vi "ILD from Array Data for S4p Tool.vi"(8 "Frequency":dbl[](array[numeric]), 9 "Data in":dbl[][](array[numeric]) caption="Data In" format="%0.3f", 10 "Data path":path caption="Data Save Path", 11 "Spec":enum16{"IEEE802.3ba", "FDR", "EDR"}(ring)) -> (1 "Data out":dbl[][](array[numeric]), 2 "ILD":cluster{"all rows":dbl[], sgl[]}[](graph), 3 "IL Fitted":cluster{"all rows":dbl[], "IL":dbl[]}[](graph))   [LabVIEW 2011]
uses:
  <vilib>/Analysis/baseanly.llb/Real A x B.vi
  <vilib>/Analysis/baseanly.llb/Real Inverse Matrix.vi
  <vilib>/Analysis/baseanly.llb/A x Vector.vi
  <vilib>/Utility/file.llb/Write To Spreadsheet File (DBL).vi
  <vilib>/Analysis/NI_AALBase.lvlib
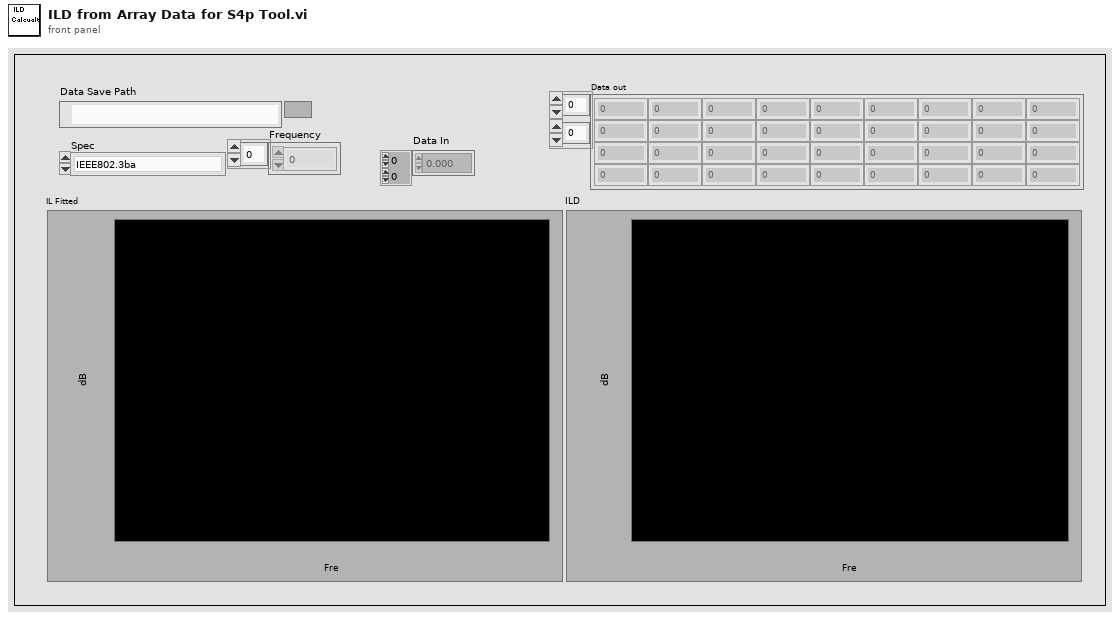
[diagram p1: front panel]
types:
  T1 = typedef "NI_Matrix.lvlib/RealMatrix.ctl" = dbl[][]
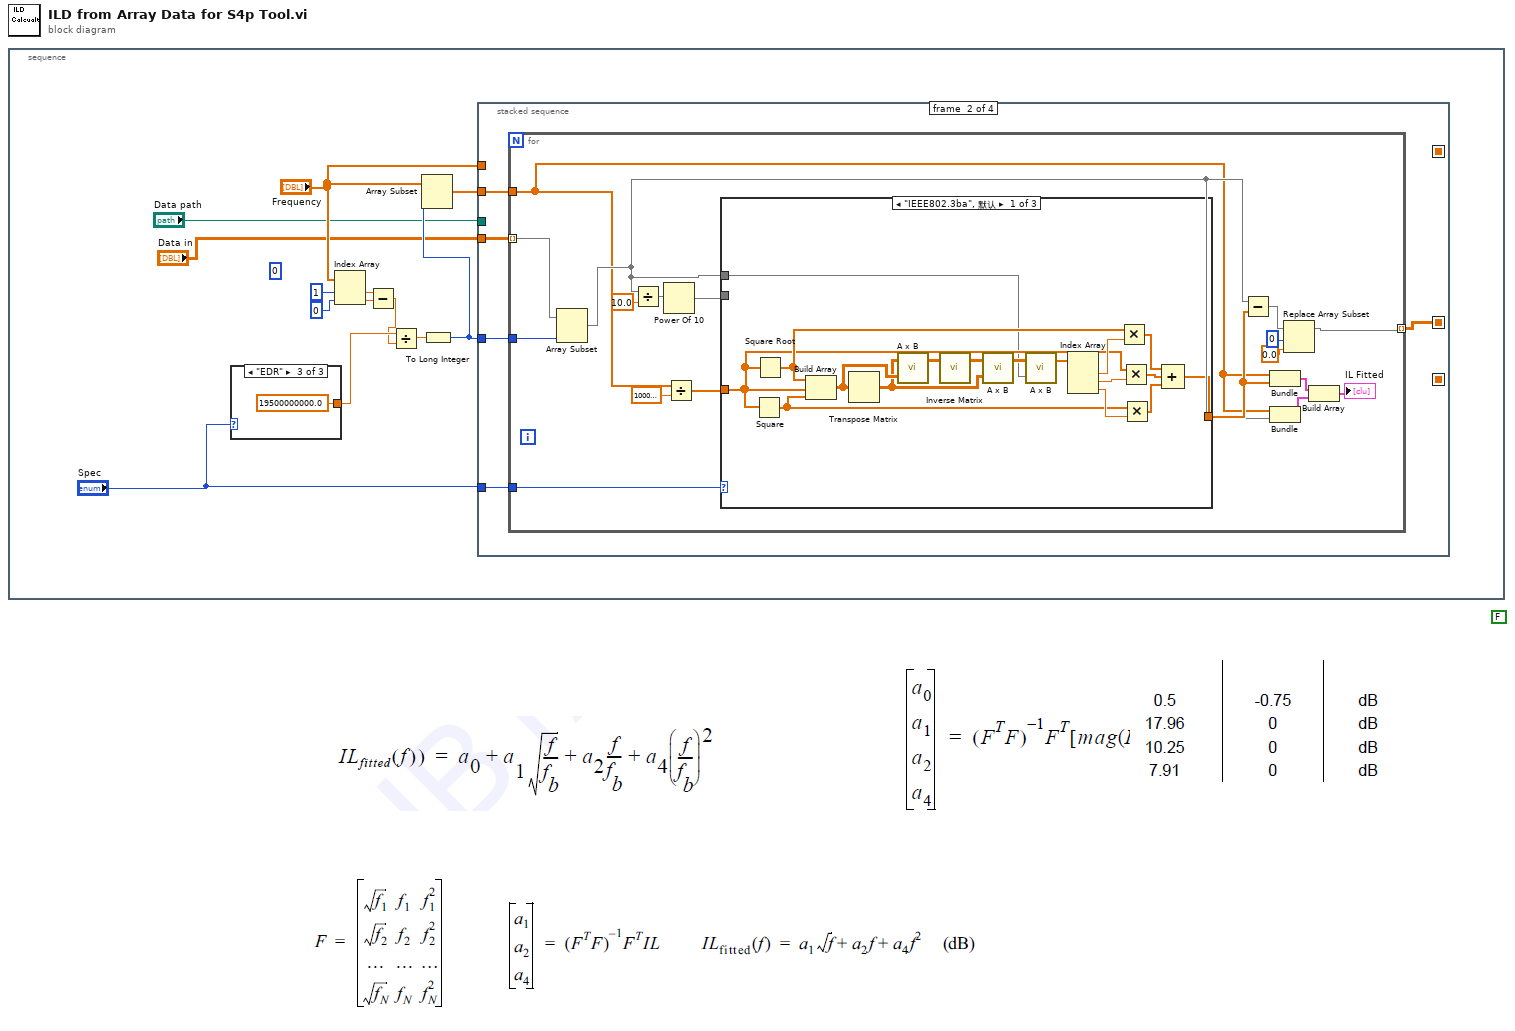
[diagram p0: block diagram]
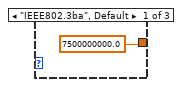
[diagram p2: hidden frame]
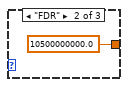
[diagram p3: hidden frame]
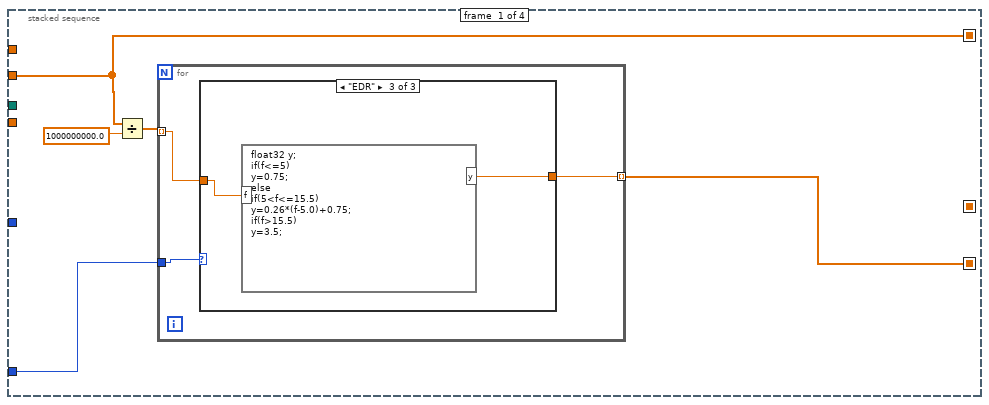
[diagram p4: hidden frame]
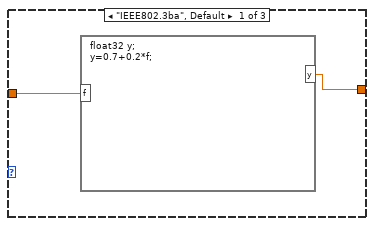
[diagram p5: hidden frame]
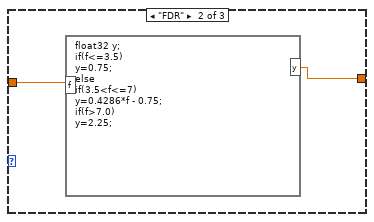
[diagram p6: hidden frame]
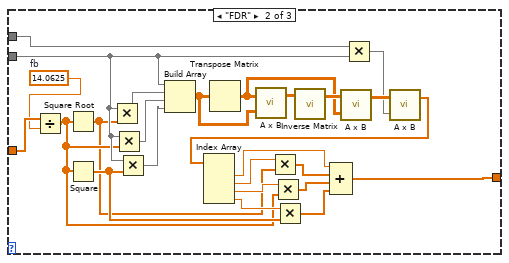
[diagram p7: hidden frame]
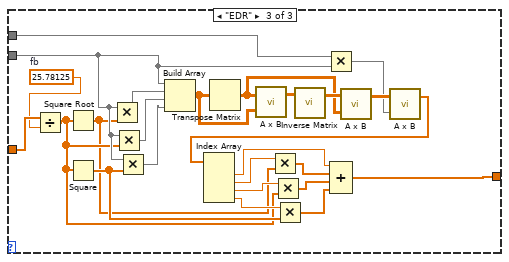
[diagram p8: hidden frame]
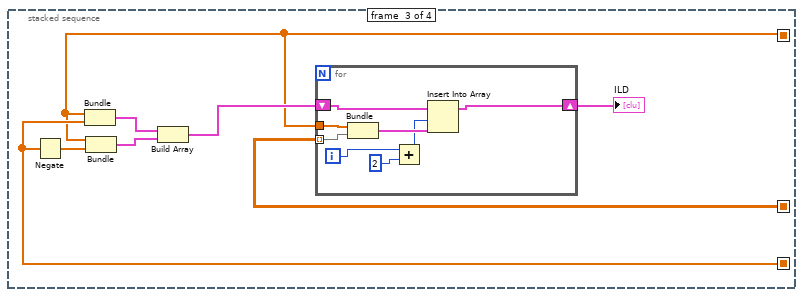
[diagram p9: hidden frame]
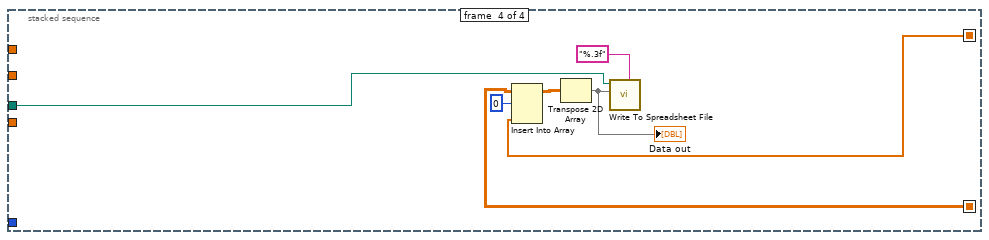
[diagram p10: hidden frame]
diagram:
  (unwired) FALSE
  n1 = stacked-sequence {
    frame #0 {
      (unwired) 0 ("禁用的索引 (列)")
      n2 = case shown="\"EDR\"" "Spec" {
        tunnel: [7500000000.0 ("y") 10500000000.0 ("y") 19500000000.0 ("y")] -> w10
        frame "IEEE802.3ba", Default {
        }
        frame "FDR" {
        }
        frame "EDR" {
        }
      }
      n3 = Index Array(array="Frequency", index #1=1 ("索引"), index #2=0 ("索引")) -> (element #1=w8:dbl, element #2=w9:dbl)
      n4 = Subtract(x=w8, y=w9) -> (x-y=w7:dbl)
      n5 = Divide(x=w10, y=w7) -> (x/y=w6:dbl)
      n6 = To Long Integer(number=w6) -> (32bit integer=w4:i32)
      n7 = Array Subset(array="Frequency", length=w4) -> (w5:dbl[])  [unwired: 1 in]
      n8 = stacked-sequence {
        seq-local: [w20 _ _ _] -> [_ _ w126 _]
        seq-local: [w17 _ _ _] -> [_ _ w122 w140]
        seq-local: [_ w33 _ _] -> [_ _ w123 w141]
        tunnel: "Data in" -> [_ w35 _ _]
        tunnel: "Spec" -> [w21 w34 _ _]
        tunnel: w5 -> [w17 w32 _ _]
        tunnel: "Data path" -> [_ _ _ w137]
        tunnel: w4 -> [_ w31 _ _]
        tunnel: "Frequency" -> [_ _ _ _]
        frame #0 {
          n9 = Divide(x=w17, y=1000000000.0) -> (x/y=w19:dbl[])
          n10 = for {
            tunnel: w21 -> [w24]
            tunnel: w19 -> [w23] mode=indexing
            tunnel: [w22] -> w20 mode=indexing
            n11 = case shown="\"EDR\"" w24 {
              tunnel: w23 -> [w26 w28 w30]
              tunnel: [w25 w27 w29] -> w22
              frame "IEEE802.3ba", Default {
                n12 = formula code="float32 y;\ny=0.7+0.2*f;"("f"=w26) -> ("y"=w25:sgl)
              }
              frame "FDR" {
                n13 = formula code="float32 y;\nif(f<=3.5)\ny=0.75;\nelse\nif(3.5<f<=7)\ny=0.4286*f - 0.75;\nif(f>7.0)\ny=2.25;"("f"=w28) -> ("y"=w27:sgl)
              }
              frame "EDR" {
                n14 = formula code="float32 y;\nif(f<=5)\ny=0.75;\nelse\nif(5<f<=15.5)\ny=0.26*(f-5.0)+0.75;\nif(f>15.5)\ny=3.5;"("f"=w30) -> ("y"=w29:sgl)
              }
            }
          }
        }
        frame #1 {
          n15 = for {
            tunnel: w35 -> [w36] mode=indexing
            tunnel: [w45] -> w33 mode=indexing
            tunnel: w34 -> [w44]
            tunnel: w32 -> [w37]
            tunnel: w31 -> [w39]
            n16 = Array Subset(array=w36, length=w39) -> (w38:dbl[])  [unwired: 1 in]
            n17 = Divide(x=w38, y=10.0 ("新元素/子数组")) -> (x/y=w42:dbl[])
            n18 = Power Of 10(x=w42) -> (10^x=w41:dbl[])
            n19 = Divide(x=w37, y=1000000000.0) -> (x/y=w40:dbl[])
            n20 = case shown="\"IEEE802.3ba\", 默认" w44 {
              tunnel: [w56 w71 w96] -> w49
              tunnel: w40 -> [w55 w95 w120]
              tunnel: w38 -> [w54 w85 w110]
              tunnel: w41 -> [_ w84 w109]
              frame "IEEE802.3ba", Default {
                n21 = Square(x=w55) -> (x^2=w60:dbl[])
                n22 = Square Root(x=w55) -> (sqrt(x)=w61:dbl[])
                n23 = Build Array(w61, w55, w60) -> (w70:T1)
                n24 = Transpose Matrix(1:w70) -> (0:w68:T1)
                n25 = call-poly <vilib>:"A x B.vi"("B"=w70, "A"=w68) -> ("A x B"=w69:T1)  [unwired: 1 out]
                n26 = call-poly <vilib>:"Inverse Matrix.vi"("Input Matrix"=w69) -> ("Inverse Matrix"=w67:T1)  [unwired: 1 in, 1 out]
                n27 = call-poly <vilib>:"A x B.vi"("B"=w68, "A"=w67) -> ("A x B"=w66:T1)  [unwired: 1 out]
                n28 = call-poly <vilib>:"A x B.vi"("Vector"=w54, "A"=w66) -> ("A x Vector"=w65:dbl[])  [unwired: 1 out]
                n29 = Index Array(array=w65) -> (element #1=w62:dbl, element #2=w63:dbl, element #3=w64:dbl)  [unwired: 3 in]
                n30 = Multiply(x=w61, y=w62) -> (x*y=w59:dbl[])
                n31 = Multiply(x=w55, y=w63) -> (x*y=w58:dbl[])
                n32 = Multiply(x=w60, y=w64) -> (x*y=w57:dbl[])
                n33 = Compound Arithmetic op=ADD(w59, w58, w57) -> (w56:dbl[])
              }
              frame "FDR" {
                w94 = 14.0625  # fb
                n34 = Divide(x=w95, y=w94) -> (x/y=w73:dbl[])
                n35 = Square Root(x=w73) -> (sqrt(x)=w72:dbl[])
                n36 = Square(x=w73) -> (x^2=w74:dbl[])
                n37 = Multiply(x=w84, y=w72) -> (x*y=w93:dbl[])
                n38 = Multiply(x=w84, y=w73) -> (x*y=w92:dbl[])
                n39 = Multiply(x=w84, y=w74) -> (x*y=w91:dbl[])
                n40 = Build Array(w84, w93, w92, w91) -> (w90:T1)
                n41 = Transpose Matrix(1:w90) -> (0:w87:T1)
                n42 = call-poly <vilib>:"A x B.vi"("B"=w90, "A"=w87) -> ("A x B"=w89:T1)  [unwired: 1 out]
                n43 = call-poly <vilib>:"Inverse Matrix.vi"("Input Matrix"=w89) -> ("Inverse Matrix"=w88:T1)  [unwired: 1 in, 1 out]
                n44 = call-poly <vilib>:"A x B.vi"("B"=w87, "A"=w88) -> ("A x B"=w86:T1)  [unwired: 1 out]
                n45 = Multiply(x=w85, y=w84) -> (x*y=w83:dbl[])
                n46 = call-poly <vilib>:"A x B.vi"("Vector"=w83, "A"=w86) -> ("A x Vector"=w82:dbl[])  [unwired: 1 out]
                n47 = Index Array(array=w82) -> (element #1=w81:dbl, element #2=w80:dbl, element #3=w79:dbl, element #4=w78:dbl)  [unwired: 4 in]
                n48 = Multiply(x=w80, y=w72) -> (x*y=w77:dbl[])
                n49 = Multiply(x=w79, y=w73) -> (x*y=w76:dbl[])
                n50 = Multiply(x=w78, y=w74) -> (x*y=w75:dbl[])
                n51 = Compound Arithmetic op=ADD(w81, w77, w76, w75) -> (w71:dbl[])
              }
              frame "EDR" {
                w119 = 25.78125  # fb
                n52 = Divide(x=w120, y=w119) -> (x/y=w98:dbl[])
                n53 = Square Root(x=w98) -> (sqrt(x)=w97:dbl[])
                n54 = Square(x=w98) -> (x^2=w99:dbl[])
                n55 = Multiply(x=w109, y=w97) -> (x*y=w118:dbl[])
                n56 = Multiply(x=w109, y=w98) -> (x*y=w117:dbl[])
                n57 = Multiply(x=w109, y=w99) -> (x*y=w116:dbl[])
                n58 = Build Array(w109, w118, w117, w116) -> (w115:T1)
                n59 = Transpose Matrix(1:w115) -> (0:w112:T1)
                n60 = call-poly <vilib>:"A x B.vi"("B"=w115, "A"=w112) -> ("A x B"=w114:T1)  [unwired: 1 out]
                n61 = call-poly <vilib>:"Inverse Matrix.vi"("Input Matrix"=w114) -> ("Inverse Matrix"=w113:T1)  [unwired: 1 in, 1 out]
                n62 = Multiply(x=w110, y=w109) -> (x*y=w108:dbl[])
                n63 = call-poly <vilib>:"A x B.vi"("B"=w112, "A"=w113) -> ("A x B"=w111:T1)  [unwired: 1 out]
                n64 = call-poly <vilib>:"A x B.vi"("Vector"=w108, "A"=w111) -> ("A x Vector"=w107:dbl[])  [unwired: 1 out]
                n65 = Index Array(array=w107) -> (element #1=w106:dbl, element #2=w105:dbl, element #3=w104:dbl, element #4=w103:dbl)  [unwired: 4 in]
                n66 = Multiply(x=w105, y=w97) -> (x*y=w102:dbl[])
                n67 = Multiply(x=w104, y=w98) -> (x*y=w101:dbl[])
                n68 = Multiply(x=w103, y=w99) -> (x*y=w100:dbl[])
                n69 = Compound Arithmetic op=ADD(w106, w102, w101, w100) -> (w96:dbl[])
              }
            }
            n70 = Subtract(x=w38, y=w49) -> (x-y=w48:dbl[])
            n71 = Bundle(w37, w49) -> (w53:cluster{dbl[], dbl[]})  [unwired: 1 in]
            n72 = Bundle(w37, w38) -> (w52:cluster{dbl[], dbl[]})  [unwired: 1 in]
            n73 = Replace Array Subset(array=w48, new element=0.0 ("新元素/子数组"), index=0 ("索引")) -> (w45:dbl[])
            n74 = Build Array(w53, w52) -> (→"IL Fitted":cluster{dbl[], dbl[]}[])
          }
        }
        frame #2 {
          n75 = Negate(x=w126) -> (-x=w127:sgl[])
          n76 = Bundle(w122, w126) -> (w125:cluster{dbl[], sgl[]})  [unwired: 1 in]
          n77 = Bundle(w122, w127) -> (w128:cluster{dbl[], sgl[]})  [unwired: 1 in]
          n78 = Build Array(w125, w128) -> (w124:cluster{dbl[], sgl[]}[])
          n79 = for {
            shift-right: [w132] -> w121
            shift-left: w124 -> [w134]
            tunnel: w123 -> [w136] mode=indexing
            tunnel: w122 -> [w135]
            i -> [w131]
            n80 = Bundle(w135, w136) -> (w133:cluster{dbl[], dbl[]})  [unwired: 1 in]
            n81 = Add(x=w131, y=2) -> (x+y=w129:i32)
            n82 = Insert Into Array(array=w134, index=w129, new element=w133) -> (w132:cluster{dbl[], sgl[]}[])
          }
          "ILD" <- w121
        }
        frame #3 {
          n83 = Insert Into Array(array=w141, index (row)=0 ("索引 (行)"), new element=w140) -> (w143:dbl[][])  [unwired: 1 in]
          n84 = Transpose 2D Array(2D array=w143) -> (transposed array=w139:dbl[][])
          "Data out" <- w139
          n85 = call-poly <vilib>:"Write To Spreadsheet File.vi"("format (%.3f)"="%.3f", "2D data"=w139, "file path (dialog if empty)"=w137) -> ()  [unwired: 5 in, 1 out]
        }
      }
    }
  }
